vi "ofdmtx2.vi"(1 "Transmitter Properties":T1 {"Window" items=["Rectangular", "Bohman", "Parzen", "Bartlett-Hanning", "Blackman-Nuttall", "Blackman", "Hanning", "Hamming", "Welch", "Exact Blackman", "Blackman-Harris", "Triangle"]}, 2 "Generate Training Symbol":bool, 3 "Input Bits":bool[](array[boolean])) -> (0 "OFDM Signal":cdb[](array[numeric]))   [LabVIEW 2013]
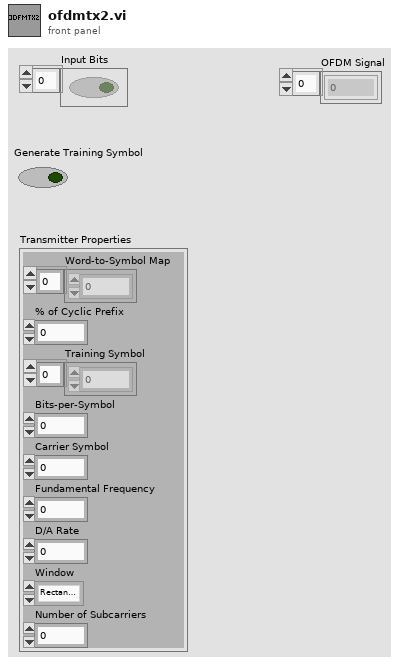
[diagram p1: front panel]
types:
  T1 = cluster{"Word-to-Symbol Map":cdb[], "% of Cyclic Prefix":dbl, "Training Symbol":cdb[], "Bits-per-Symbol":i32, "Carrier Symbol":cdb, "Fundamental Frequency":dbl, "D/A Rate":dbl, "Window":u16, "Number of Subcarriers":i32}
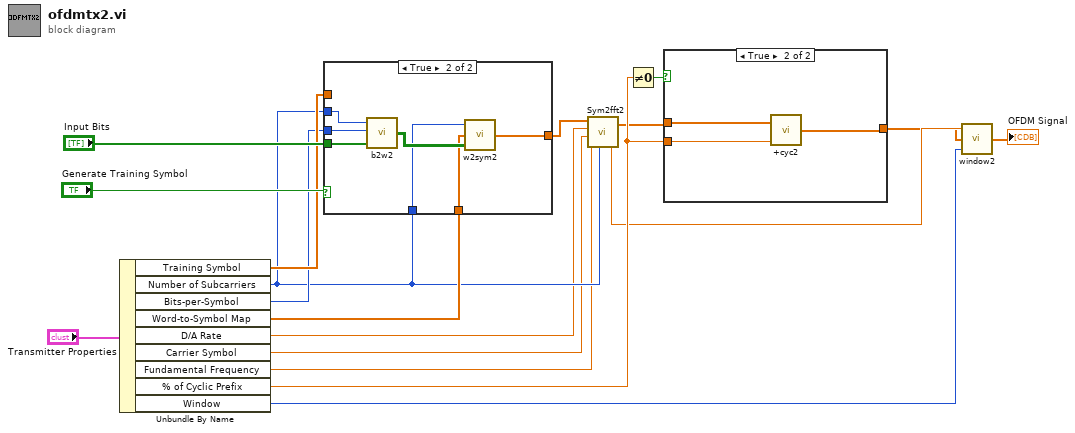
[diagram p0: block diagram]
diagram:
  n1 = Unbundle By Name("Transmitter Properties") -> ("Training Symbol"=w15:cdb[], "Number of Subcarriers"=w11:i32, "Bits-per-Symbol"=w14:i32, "Word-to-Symbol Map"=w12:cdb[], "D/A Rate"=w10:dbl, "Carrier Symbol"=w9:cdb, "Fundamental Frequency"=w8:dbl, "% of Cyclic Prefix"=w5:dbl, "Window"=w7:u16)
  n2 = case shown="True" "Generate Training Symbol" {
    tunnel: "Input Bits" -> [_ w26]
    tunnel: w15 -> [w19 _]
    tunnel: w14 -> [_ w25]
    tunnel: w11 -> [_ w24]
    tunnel: [w19 w22] -> w13
    tunnel: w12 -> [_ w21]
    tunnel: w11 -> [_ w20]
    frame False {
    }
    frame True {
      n3 = call "b2w2.vi"("parrel input"=w26, "bits-per-symbol"=w25, "number of subcarriers"=w24) -> ("output array"=w23:bool[][])
      n4 = call "w2sym2.vi"("Parallel Word Input"=w23, "Word-to-Symbol Map"=w21, "Number of Subcarriers"=w20) -> ("Parallel Symbol Output"=w22:cdb[])
    }
  }
  n5 = call "Sym2fft2.vi"("Parallel Symbol In"=w13, "D/A Rate"=w10, "Carrier Symbol"=w9, "Fundamental Frequency"=w8, "Number of Subcarriers"=w11) -> ("Time Domain Out"=w3:cdb[], "DC Offset"=w4:cdb)
  n6 = Not Equal To 0?(x=w5) -> (x != 0?=w6:bool)
  n7 = case shown="True" w6 {
    tunnel: w5 -> [_ w30]
    tunnel: w3 -> [w27 w29]
    tunnel: [w27 w28] -> w2
    frame False {
    }
    frame True {
      n8 = call "+cyc2.vi"("% of Cyclic Prefix"=w30, "Original Signal"=w29) -> ("Prefixed Signal"=w28:cdb[])
    }
  }
  n9 = call "window2.vi"("Window"=w7, "Unfiltered Signal"=w2, "DC Offset"=w4) -> ("Windowed Signal"=→"OFDM Signal":cdb[])
